vi "Get APU Characteristics.vi"(8 "error in (no error)":errorcluster, 11 "Item Ref in":T1 format="%.0x") -> (0 "error out":errorcluster, 1 "angle to u16 scale factor":dbl, 2 "total angle span (degrees)":u16, 3 "Item Ref out":T1 format="%.0x", 4 "start angle":dbl, 5 "degrees of one u16":dbl, 7 "rotations":u16)   [LabVIEW 2015, in "Engine Simulation Toolkit System Explorer.lvlib"]
uses:
  Engine Simulation Toolkit System Explorer.lvlib
  <vilib>/NI Veristand/Custom Device API/Custom Device Item Ref.ctl
  <vilib>/NI Veristand/Custom Device Tools/Custom Device Utility Library/Search Direction.ctl
  Shared/Properties.vi
  Shared/Constants and GUIDs.vi
  <vilib>/NI Veristand/Custom Device Tools/Custom Device Utility Library/NI VeriStand - Search for Item by GUID.vi
  <vilib>/NI Veristand/Custom Device API/Get Item Property (U16).vi
  <vilib>/NI Veristand/Custom Device API/Get Item Property (Double).vi
  <vilib>/NI Veristand/Custom Device API/Custom Device API.lvlib
  Shared/Engine Simulation Toolkit Shared.lvlib
  <vilib>/NI Veristand/Custom Device Tools/Custom Device Utility Library/Custom Device Utility Library.lvlib
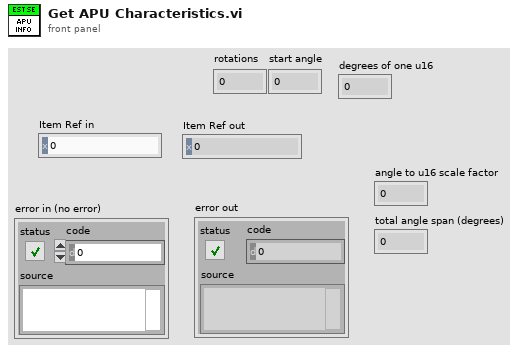
[diagram p1: front panel]
types:
  T1 = typedef "Custom Device API.lvlib/Custom Device Item Ref.ctl" = u64
  T2 = typedef "Custom Device Utility Library.lvlib/Search Direction.ctl" = enum16{"Down", "Up"}
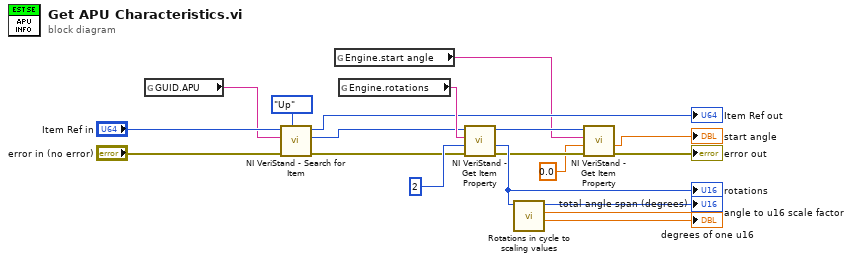
[diagram p0: block diagram]
diagram:
  n1 = global read "Constants and GUIDs.vi" "GUID.APU"() -> (w13:string)
  n2 = call-poly <vilib>:"NI VeriStand - Search for Item.vi"("Direction (Down)"=Search_Direction."Up", "error in"="error in (no error)", "Item GUID"=w13, "Section Ref in"="Item Ref in") -> ("error out"=w15:errorcluster, "Item Ref"=w12:T1, "Section Ref out"=→"Item Ref out":T1)  [unwired: 4 in, 1 out]
  n3 = global read "Properties.vi" "Engine.start angle"() -> (w3:string)
  n4 = global read "Properties.vi" "Engine.rotations"() -> (w19:string)
  n5 = call-poly <vilib>:"NI VeriStand - Get Item Property.vi"("error in (no error)"=w15, "Default Value"=u16 2, "Property Name"=w19, "Item Ref in"=w12) -> ("error out"=w9:errorcluster, "Value"=w17:u16, "Item Ref out"=w4:T1)  [unwired: 4 in, 1 out]
  "rotations" <- w17
  n6 = call "Rotations in cycle to scaling values.vi"("rotations in a cycle"=w17) -> ("degrees of one u16"=→"degrees of one u16":dbl, "angle to u16 scale factor"=→"angle to u16 scale factor":dbl, "total angle span (degrees)"=→"total angle span (degrees)":u16)  [unwired: 8 in]
  n7 = call-poly <vilib>:"NI VeriStand - Get Item Property.vi"("error in (no error)"=w9, "Default Value"=0.0, "Property Name"=w3, "Item Ref in"=w4) -> ("error out"=→"error out":errorcluster, "Value"=→"start angle":dbl)  [unwired: 4 in, 2 out]
